vi "Start Probe FP.vi"(8 "error in (no error)":errorcluster, 10 "Cached Probe vi path":path, 11 "Refnums":i32[](array[numeric])) -> (0 "error out":errorcluster, 3 "Probe VI":refnum<vi>)   [LabVIEW 2019, in "GOOP Probe.lvlib"]
uses:
  GOOP Probe.lvlib
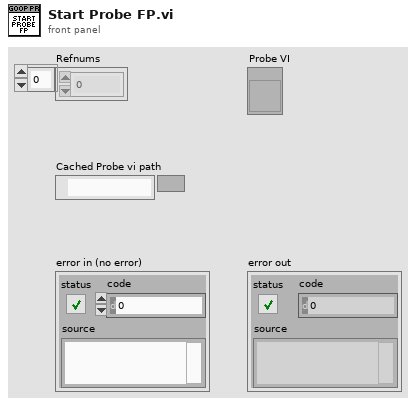
[diagram p1: front panel]
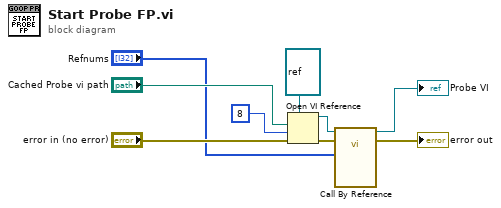
[diagram p0: block diagram]
diagram:
  n1 = Open VI Reference(type specifier VI Refnum (for type only)=refnum<vi> refnum, vi path="Cached Probe vi path", options=8, error in (no error)="error in (no error)") -> (vi reference=w5:refnum<vi>, error out=w6:errorcluster)  [unwired: 2 in]
  n2 = call-by-ref "?"(reference=w5, error in=w6, "Refs"="Refnums") -> (reference out=→"Probe VI":refnum<vi>, error out=→"error out":errorcluster)  [unwired: 11 in]
